vi "Teleop.vi"(10 "Match Info":T1={"Autonomous Elapsed Seconds"=0.0, "TeleOp Elapsed Seconds"=0.0, "Disabled Elapsed Seconds"=0.0, "Visited Autonomous"=FALSE, "Visited TeleOp"=FALSE, "Visited Disabled"=FALSE, "Autonomous Settings"={"Autonomous Style"=enum."Independent", "VI Refnum"=refnum}}, 11 "Call Context":T2) -> ()   [LabVIEW 2013]
doc: "This VI is called for each TeleOp packet received from the DS where the robot is not disabled. It is often used to read from the joysticks and update I/O or to update setpoints for timed control loops. It should complete and return within 20 milliseconds or it may miss DS packets."
uses:
  <vilib>/Rock Robotics/WPI/DriverStation/WPI_DriverStationDerivedRobotMode.ctl
  <vilib>/Rock Robotics/WPI/DriverStation/WPI_DriverStationMatch Info.ctl
  <vilib>/Rock Robotics/WPI/Relay/WPI_RelayValue.ctl
  <vilib>/Rock Robotics/WPI/Solenoid/WPI_SolenoidValue.ctl
  Robot Global Data.vi
  <vilib>/Rock Robotics/WPI/Joystick/WPI_JoystickGetSetRefNum.vi
  <vilib>/Rock Robotics/WPI/Solenoid/WPI_SolenoidSetEnum.vi
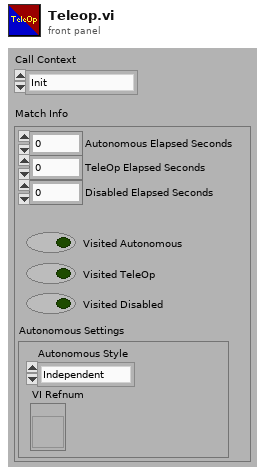
[diagram p1: front panel]
types:
  T1 = typedef "WPI_DriverStationMatch Info.ctl" = cluster{"Autonomous Elapsed Seconds":dbl, "TeleOp Elapsed Seconds":dbl, "Disabled Elapsed Seconds":dbl, "Visited Autonomous":bool, "Visited TeleOp":bool, "Visited Disabled":bool, "Autonomous Settings":cluster{"Autonomous Style":enum16{"Iterative", "Independent"}, "VI Refnum":refnum<vi>}}
  T2 = typedef "WPI_DriverStationDerivedRobotMode.ctl" = enum16{"Init", "Execute", "Stop"}
  T3 = typedef "WPI_RelayValue.ctl" = enum16{"Off", "On", "Forward", "Reverse"}
  T4 = typedef "WPI_JoystickDevRef.ctl" = cluster{"Device":T5}
  T5 = typedef "WPI_JoystickDeviceEnum.ctl" = enum16{"USB 1", "USB 2", "USB 3", "USB 4", "Kinect 1", "Kinect 2"}
  T6 = typedef "WPI_JoystickButtonState.ctl" = cluster{"Button 1":bool, "Button 2":bool, "Button 3":bool, "Button 4":bool, "Button 5":bool, "Button 6":bool, "Button 7":bool, "Button 8":bool, "Button 9":bool, "Button 10":bool, "Button 11":bool, "Button 12":bool}
  T7 = cluster{"axis 1 (x)":dbl, "axis 2 (y)":dbl, "axis 3 (throttle)":dbl, "axis 4":dbl, "axis 5":dbl, "axis 6":dbl}
  T8 = typedef "WPI_RelayDevRef.ctl" = cluster{"DevStatus":errorcluster, "Relay Channel":T9, "Digital Module":T10, "Relay Direction":T11}
  T9 = typedef "FPGA_DIORelayChannel.ctl" = enum8{"Relay 1", "Relay 2", "Relay 3", "Relay 4", "Relay 5", "Relay 6", "Relay 7", "Relay 8", "Invalid"}
  T10 = typedef "FPGA_TypedefDigitalModule.ctl" = enum16{"Digital Module 1", "Digital Module 2"}
  T11 = typedef "WPI_RelayDirection.ctl" = enum16{"Both directions", "Forward only", "Reverse only"}
  T12 = typedef "WPI_ServoDeviceRef.ctl" = cluster{"DeviceStatus":errorcluster, "Digital Module":T10, "PWM Channel":T13, "DeadBand":T14}
  T13 = typedef "FPGA_DIOPWMChannel.ctl" = enum8{"PWM 1", "PWM 2", "PWM 3", "PWM 4", "PWM 5", "PWM 6", "PWM 7", "PWM 8", "PWM 9", "PWM 10", "Invalid"}
  T14 = typedef "WPI_PWMDeadband.ctl" = cluster{"Name":string, "maxPositivePwm":i32, "minPositivePwm":i32, "centerPwm":i32, "maxNegativePwm":i32, "minNegativePwm":i32, "angularRange":u16}
  T15 = typedef "WPI_SolenoidValue.ctl" = enum16{"Off", "On", "Forward", "Reverse"}
  T16 = typedef "WPI_SolenoidDevRef.ctl" = cluster{"DevStatus":errorcluster, "Solenoid Module":T17, "Forward Solenoid Channel":T18, "Reverse Solenoid Channel":T18}
  T17 = typedef "FPGA_TypedefSolenoidModule.ctl" = enum16{"Solenoid Module 1", "Solenoid Module 2"}
  T18 = typedef "WPI_SolenoidChannel.ctl" = enum8{"Solenoid 1", "Solenoid 2", "Solenoid 3", "Solenoid 4", "Solenoid 5", "Solenoid 6", "Solenoid 7", "Solenoid 8", "Invalid"}
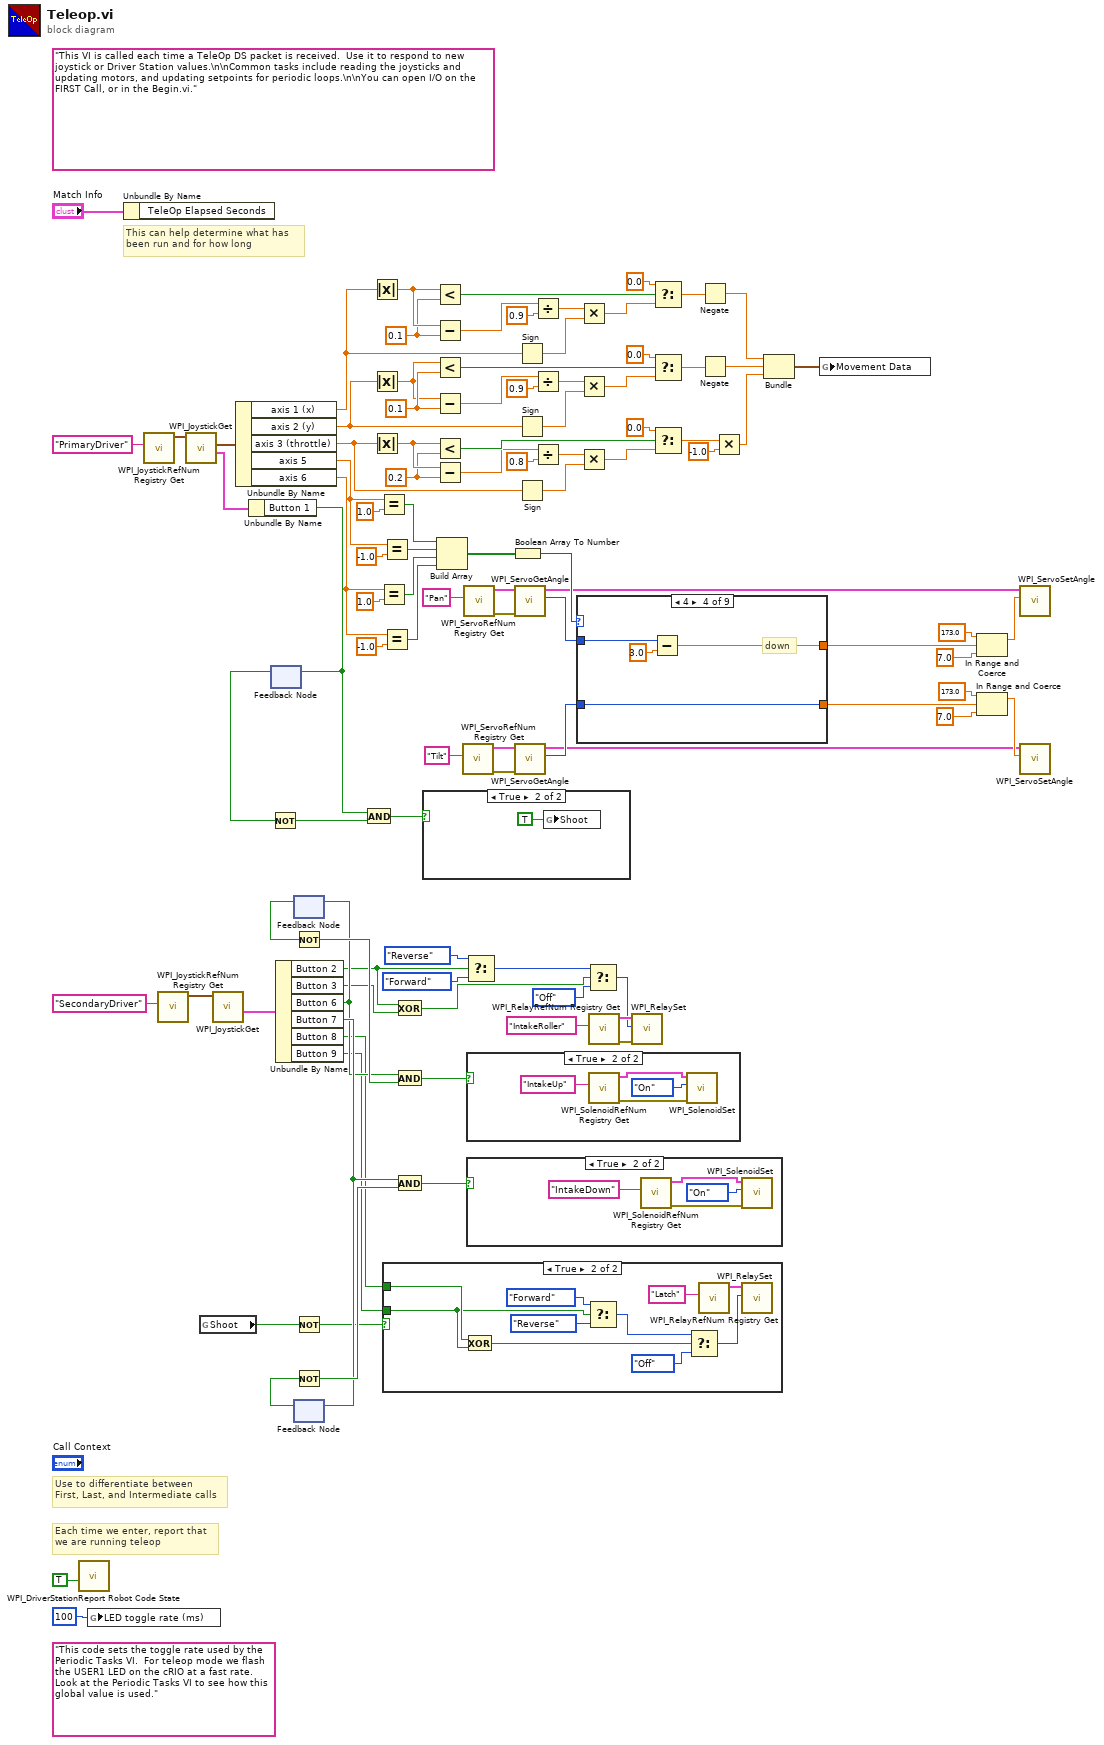
[diagram p0: block diagram]
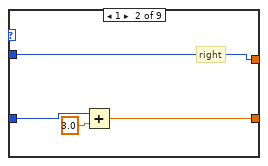
[diagram p4: hidden frame]
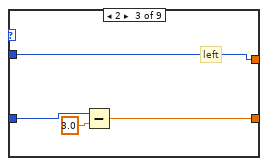
[diagram p5: hidden frame]
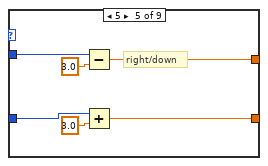
[diagram p6: hidden frame]
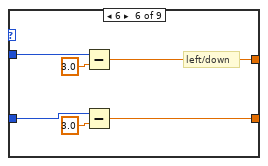
[diagram p7: hidden frame]
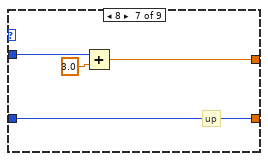
[diagram p8: hidden frame]
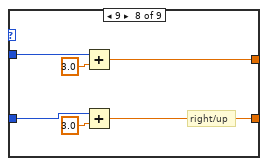
[diagram p9: hidden frame]
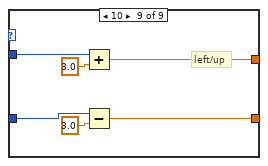
[diagram p10: hidden frame]
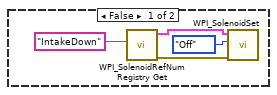
[diagram p11: hidden frame]
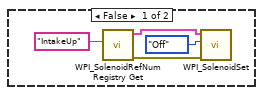
[diagram p12: hidden frame]
diagram:
  w70 = 0.2 ("y")
  w77 = 0.1 ("y")
  w91 = 0.1 ("y")
  (unwired) "This code sets the toggle rate used by the Periodic Tasks VI.  For teleop mode we flash the USER1 LED on the cRIO at a fast rate.  Look at the Periodic Tasks VI to see how this global value is used."
  (unwired) "This VI is called each time a TeleOp DS packet is received.  Use it to respond to new joystick or Driver Station values.\n\nCommon tasks include reading the joysticks and updating motors, and updating setpoints for periodic loops.\n\nYou can open I/O on the FIRST Call, or in the Begin.vi."
  # "Each time we enter, report that\nwe are running teleop"
  # "Use to differentiate between\nFirst, Last, and Intermediate calls"
  # "This can help determine what has\nbeen run and for how long"
  n1 = call <vilib>:"WPI_DriverStationReport Robot Code State.vi"("TeleOp"=TRUE ("Autonomous")) -> ()  [unwired: 10 in, 1 out]
  n2 = global write "Robot Global Data.vi" "LED toggle rate (ms)"(u32 100 ("LED ms toggle rate")) -> ()
  n3 = Unbundle By Name("Match Info") -> ()  [unwired: 1 out]
  n4 = call <vilib>:"WPI_JoystickRefNum Registry Get.vi"("refnum name"="PrimaryDriver") -> ("JoystickDevRef"=w102:T4)  [unwired: 9 in, 1 out]
  n5 = call <vilib>:"WPI_JoystickRefNum Registry Get.vi"("refnum name"="SecondaryDriver") -> ("JoystickDevRef"=w55:T4)  [unwired: 9 in, 1 out]
  n6 = call <vilib>:"WPI_JoystickGet.vi"("JoystickDevRef"=w102) -> ("Buttons"=w99:T6, "Axes"=w100:T7)  [unwired: 4 in, 1 out]
  n7 = global read "Robot Global Data.vi" "Shoot"() -> (w4:bool)
  n8 = call <vilib>:"WPI_JoystickGet.vi"("JoystickDevRef"=w55) -> ("Buttons"=w54:T6)  [unwired: 4 in, 2 out]
  n9 = Unbundle By Name(w100) -> ("axis 1 (x)"=w87:dbl, "axis 2 (y)"=w64:dbl, "axis 3 (throttle)"=w63:dbl, "axis 5"=w34:dbl, "axis 6"=w33:dbl)
  n10 = Unbundle By Name(w99) -> ("Button 1"=w97:bool)
  n11 = feedback-in #1(w97) -> ()
  n12 = feedback #1() -> (w96:bool)  [unwired: 1 in]
  n13 = Not(x=w96) -> (.not. x?=w95:bool)
  n14 = Unbundle By Name(w54) -> ("Button 2"=w42:bool, "Button 3"=w45:bool, "Button 6"=w47:bool, "Button 7"=w51:bool, "Button 8"=w2:bool, "Button 9"=w1:bool)
  n15 = feedback #2() -> (w48:bool)  [unwired: 1 in]
  n16 = feedback-in #2(w47) -> ()
  n17 = Not(x=w48) -> (.not. x?=w49:bool)
  n18 = Not(x=w4) -> (.not. x?=w3:bool)
  n19 = feedback #3() -> (w52:bool)  [unwired: 1 in]
  n20 = Not(x=w52) -> (.not. x?=w53:bool)
  n21 = feedback-in #3(w51) -> ()
  n22 = And(x=w97, y=w95) -> (x .and. y?=w98:bool)
  n23 = Absolute Value(x=w87) -> (abs(x)=w92:dbl)
  n24 = Absolute Value(x=w64) -> (abs(x)=w76:dbl)
  n25 = Absolute Value(x=w63) -> (abs(x)=w71:dbl)
  n26 = Equal?(x=w34, y=1.0) -> (x = y?=w28:bool)
  n27 = Equal?(x=w33, y=1.0) -> (x = y?=w26:bool)
  n28 = Equal?(x=w34, y=-1.0) -> (x = y?=w27:bool)
  n29 = Equal?(x=w33, y=-1.0) -> (x = y?=w25:bool)
  n30 = case shown="True" w3 {
    tunnel: w2 -> [_ w107]
    tunnel: w1 -> [_ w106]
    frame False {
    }
    frame True {
      n31 = Exclusive Or(1:w106, 2:w107) -> (0:w108:bool)
      n32 = Select(t=WPI_RelayValue."Forward" ("RelayValue"), s=w106, f=WPI_RelayValue."Reverse" ("RelayValue")) -> (s? t:f=w113:T3)
      n33 = Select(t=w113, s=w108, f=WPI_RelayValue."Off") -> (s? t:f=w109:T3)
      n34 = call <vilib>:"WPI_RelayRefNum Registry Get.vi"("refnum name"="Latch") -> ("RelayDevRef"=w110:T8)  [unwired: 9 in, 1 out]
      n35 = call <vilib>:"WPI_RelaySet.vi"("RelayValue"=w109, "RelayDevRef"=w110) -> ()  [unwired: 8 in, 2 out]
    }
  }
  n36 = Exclusive Or(1:w45, 2:w42) -> (0:w43:bool)
  n37 = And(x=w47, y=w49) -> (x .and. y?=w46:bool)
  n38 = And(x=w51, y=w53) -> (x .and. y?=w50:bool)
  n39 = case shown="True" w98 {
    frame False {
    }
    frame True {
      n40 = global write "Robot Global Data.vi" "Shoot"(TRUE ("Shoot")) -> ()
    }
  }
  n41 = Less?(x=w92, y=w91) -> (x < y?=w93:bool)
  n42 = Subtract(x=w92, y=w91) -> (x-y=w90:dbl)
  n43 = Less?(x=w76, y=w77) -> (x < y?=w75:bool)
  n44 = Subtract(x=w76, y=w77) -> (x-y=w78:dbl)
  n45 = Less?(x=w71, y=w70) -> (x < y?=w72:bool)
  n46 = Subtract(x=w71, y=w70) -> (x-y=w69:dbl)
  n47 = Build Array(w28, w27, w26, w25) -> (w24:bool[])
  n48 = call <vilib>:"WPI_ServoRefNum Registry Get.vi"("refnum name"="Tilt") -> ("error out"=w20:errorcluster, "ServoDeviceRef"=w19:T12)  [unwired: 9 in]
  n49 = call <vilib>:"WPI_ServoRefNum Registry Get.vi"("refnum name"="Pan") -> ("error out"=w21:errorcluster, "ServoDeviceRef"=w22:T12)  [unwired: 9 in]
  n50 = Select(t=WPI_RelayValue."Reverse" ("RelayValue"), s=w42, f=WPI_RelayValue."Forward" ("RelayValue")) -> (s? t:f=w41:T3)
  n51 = case shown="True" w46 {
    frame False {
      n52 = call <vilib>:"WPI_SolenoidRefNum Registry Get.vi"("refnum name"="IntakeUp") -> ("error out"=w120:errorcluster, "SolenoidDevRef"=w119:T16)  [unwired: 9 in]
      n53 = call-poly <vilib>:"WPI_SolenoidSet.vi"("error in (no error)"=w120, "Value"=WPI_SolenoidValue."Off", "SolenoidDevRef"=w119) -> ()  [unwired: 7 in, 2 out]
    }
    frame True {
      n54 = call <vilib>:"WPI_SolenoidRefNum Registry Get.vi"("refnum name"="IntakeUp") -> ("error out"=w124:errorcluster, "SolenoidDevRef"=w123:T16)  [unwired: 9 in]
      n55 = call-poly <vilib>:"WPI_SolenoidSet.vi"("error in (no error)"=w124, "Value"=WPI_SolenoidValue."On", "SolenoidDevRef"=w123) -> ()  [unwired: 7 in, 2 out]
    }
  }
  n56 = case shown="True" w50 {
    frame False {
      n57 = call <vilib>:"WPI_SolenoidRefNum Registry Get.vi"("refnum name"="IntakeDown") -> ("error out"=w128:errorcluster, "SolenoidDevRef"=w127:T16)  [unwired: 9 in]
      n58 = call-poly <vilib>:"WPI_SolenoidSet.vi"("error in (no error)"=w128, "Value"=WPI_SolenoidValue."Off", "SolenoidDevRef"=w127) -> ()  [unwired: 7 in, 2 out]
    }
    frame True {
      n59 = call <vilib>:"WPI_SolenoidRefNum Registry Get.vi"("refnum name"="IntakeDown") -> ("error out"=w132:errorcluster, "SolenoidDevRef"=w131:T16)  [unwired: 9 in]
      n60 = call-poly <vilib>:"WPI_SolenoidSet.vi"("error in (no error)"=w132, "Value"=WPI_SolenoidValue."On", "SolenoidDevRef"=w131) -> ()  [unwired: 7 in, 2 out]
    }
  }
  n61 = Boolean Array To Number(Boolean array=w24) -> (number=w23:u32)
  n62 = call <vilib>:"WPI_ServoGetAngle.vi"("ServoDeviceRef"=w22, "error in (no error)"=w21) -> ("ServoDeviceRef"=w7:T12, "Angle"=w18:u16)  [unwired: 6 in, 1 out]
  n63 = call <vilib>:"WPI_ServoGetAngle.vi"("ServoDeviceRef"=w19, "error in (no error)"=w20) -> ("ServoDeviceRef"=w8:T12, "Angle"=w17:u16)  [unwired: 6 in, 1 out]
  n64 = Sign(1:w87) -> (0:w86:dbl)
  n65 = Sign(1:w64) -> (0:w81:dbl)
  n66 = Sign(1:w63) -> (0:w67:dbl)
  n67 = Divide(x=w90, y=0.9) -> (x/y=w85:dbl)
  n68 = Divide(x=w78, y=0.9) -> (x/y=w82:dbl)
  n69 = Divide(x=w69, y=0.8) -> (x/y=w66:dbl)
  n70 = case shown="4" w23 {
    tunnel: w18 -> [w134 w135 w139 w145 w150 w153 w161 w164 w170]
    tunnel: [w134 w135 w139 w143 w148 w154 w159 w163 w169] -> w12
    tunnel: w17 -> [w133 w138 w142 w146 w152 w156 w162 w168 w174]
    tunnel: [w133 w136 w140 w146 w147 w155 w162 w166 w172] -> w10
    frame 0, Default {
      # "neutral"
    }
    frame 1 {
      # "right"
      n71 = Add(x=w138, y=3.0) -> (x+y=w136:dbl)
    }
    frame 2 {
      # "left"
      n72 = Subtract(x=w142, y=3.0) -> (x-y=w140:dbl)
    }
    frame 4 {
      # "down"
      n73 = Subtract(x=w145, y=3.0) -> (x-y=w143:dbl)
    }
    frame 5 {
      # "right/down"
      n74 = Subtract(x=w150, y=3.0) -> (x-y=w148:dbl)
      n75 = Add(x=w152, y=3.0) -> (x+y=w147:dbl)
    }
    frame 6 {
      # "left/down"
      n76 = Subtract(x=w153, y=3.0) -> (x-y=w154:dbl)
      n77 = Subtract(x=w156, y=3.0) -> (x-y=w155:dbl)
    }
    frame 8 {
      # "up"
      n78 = Add(x=w161, y=3.0) -> (x+y=w159:dbl)
    }
    frame 9 {
      # "right/up"
      n79 = Add(x=w164, y=3.0) -> (x+y=w163:dbl)
      n80 = Add(x=w168, y=3.0) -> (x+y=w166:dbl)
    }
    frame 10 {
      # "left/up"
      n81 = Add(x=w170, y=3.0) -> (x+y=w169:dbl)
      n82 = Subtract(x=w174, y=3.0) -> (x-y=w172:dbl)
    }
  }
  n83 = Multiply(x=w85, y=w86) -> (x*y=w84:dbl)
  n84 = Multiply(x=w82, y=w81) -> (x*y=w83:dbl)
  n85 = Multiply(x=w66, y=w67) -> (x*y=w65:dbl)
  n86 = Select(t=w41, s=w43, f=WPI_RelayValue."Off" ("RelayValue")) -> (s? t:f=w35:T3)
  n87 = call <vilib>:"WPI_RelayRefNum Registry Get.vi"("refnum name"="IntakeRoller") -> ("error out"=w36:errorcluster, "RelayDevRef"=w37:T8)  [unwired: 9 in]
  n88 = call <vilib>:"WPI_RelaySet.vi"("error in (no error)"=w36, "RelayValue"=w35, "RelayDevRef"=w37) -> ()  [unwired: 7 in, 2 out]
  n89 = Select(t=0.0, s=w93, f=w84) -> (s? t:f=w88:dbl)
  n90 = Select(t=0.0, s=w75, f=w83) -> (s? t:f=w80:dbl)
  n91 = Select(t=0.0, s=w72, f=w65) -> (s? t:f=w59:dbl)
  n92 = Negate(x=w88) -> (-x=w61:dbl)
  n93 = Negate(x=w80) -> (-x=w60:dbl)
  n94 = Multiply(x=w59, y=-1.0) -> (x*y=w57:dbl)
  n95 = Bundle(w61, w60, w57) -> (w62:cluster{dbl, dbl, dbl})  [unwired: 1 in]
  n96 = global write "Robot Global Data.vi" "Movement Data"(w62) -> ()
  n97 = In Range and Coerce(upper limit=173.0, x=w12, lower limit=7.0) -> (coerced(x)=w16:dbl)  [unwired: 1 out]
  n98 = In Range and Coerce(upper limit=173.0, x=w10, lower limit=7.0) -> (coerced(x)=w15:dbl)  [unwired: 1 out]
  n99 = call <vilib>:"WPI_ServoSetAngle.vi"("Angle"=w16, "ServoDeviceRef"=w7) -> ()  [unwired: 8 in, 2 out]
  n100 = call <vilib>:"WPI_ServoSetAngle.vi"("Angle"=w15, "ServoDeviceRef"=w8) -> ()  [unwired: 8 in, 2 out]
